vi "get_colum_from_xl_reprort.vi"(1 "colum_num":i32, 2 "report out":refnum<class "NI_report.lvclass">) -> (0 "Array":string[](array[string]))   [LabVIEW 2014]
uses:
  <vilib>/Utility/NIReport.llb/NI_report.lvclass
  <vilib>/addons/_office/excel.llb/Excel Get Data (str).vi
  <vilib>/addons/_office/NI_ReportGenerationToolkit.lvlib
  <vilib>/Utility/NIReport.llb/Excel/NI_Excel.lvclass
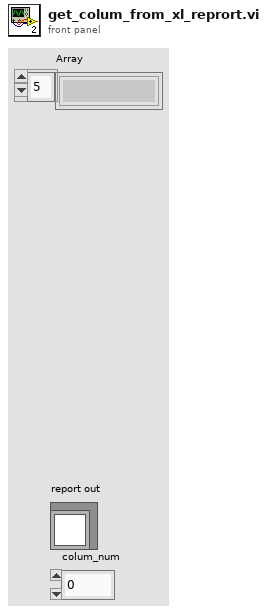
[diagram p1: front panel]
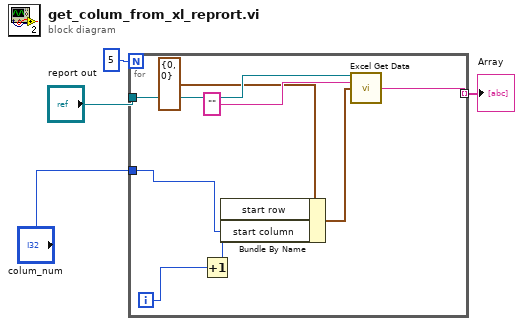
[diagram p0: block diagram]
diagram:
  n1 = for {
    N: 5 -> [_]
    tunnel: "report out" -> [w12]
    tunnel: [w8] -> w3 mode=indexing
    tunnel: "colum_num" -> [w7]
    i -> [w5]
    n2 = Increment(x=w5) -> (x+1=w6:i32)
    n3 = Bundle By Name(cluster=cluster{"start row":i32, "start column":i32} {"start row"=0, "start column"=0} ("start (0, 0)"), "start row"=w6, "start column"=w7) -> (w9:cluster{"start row":i32, "start column":i32})
    n4 = call-poly <vilib>:"Excel Get Data.vi"("report in"=w12, "data type"="", "start (0, 0)"=w9) -> ("data"=w8:string)  [unwired: 10 in, 2 out]
  }
  "Array" <- w3
